vi "PLC-Connection Status.vi"(8 "error in (no error)":errorcluster, 9 "Remarks":string, 10 "Status":bool, 11 "Controller in":refnum<class "Controller.lvclass">) -> (0 "error out":errorcluster, 3 "Controller out":refnum<class "Controller.lvclass">)   [LabVIEW 2021, in "Controller.lvlib" / "Controller.lvclass"]
uses:
  Controller.lvclass
  UserInterface/UserInterface Messages/PLC Status Msg/PLC Status Msg.lvclass
  UserInterface/UserInterface Messages/Log Data Msg/Log Data Msg.lvclass
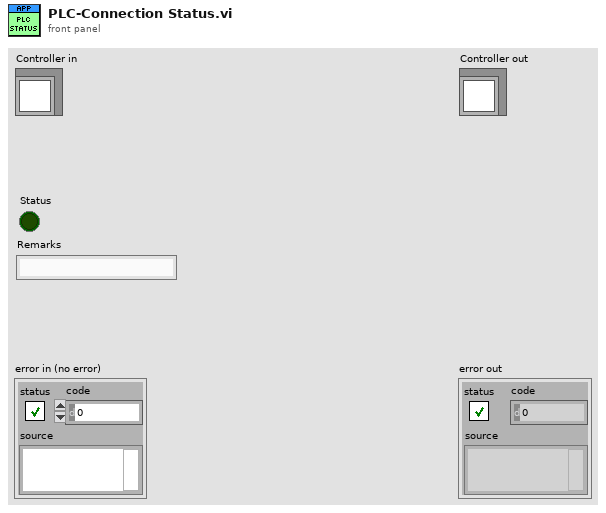
[diagram p1: front panel]
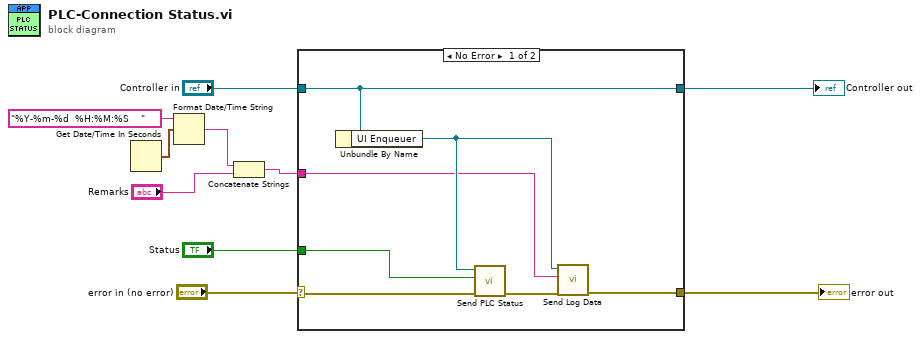
[diagram p0: block diagram]
diagram:
  n1 = Get Date/Time In Seconds() -> (seconds since 1Jan1904=w2:timestamp)
  n2 = Format Date/Time String(time format string (%c)="%Y-%m-%d  %H:%M:%S    ", seconds (now)=w2) -> (date/time string=w1:string)  [unwired: 1 in]
  n3 = Concatenate Strings(w1, "Remarks") -> (w4:string)
  n4 = case shown="No Error" "error in (no error)" {
    selector: "error in (no error)" -> [w13 w18]
    tunnel: [w17 w18] -> w10
    tunnel: "Controller in" -> [w11 w19]
    tunnel: "Status" -> [w16 _]
    tunnel: w4 -> [w12 _]
    tunnel: [w11 w19] -> w5
    frame No Error {
      n5 = Unbundle By Name(w11) -> ("UI Enqueuer"=w14:refnum<class "Message Enqueuer.lvclass">)
      n6 = call "Send PLC Status.vi"("error in (no error)"=w13, "PLC Status"=w16, "Message Enqueuer"=w14) -> ("error out"=w15:errorcluster)  [unwired: 7 in, 1 out]
      n7 = call "Send Log Data.vi"("error in (no error)"=w15, "Message"=w12, "Message Enqueuer"=w14) -> ("error out"=w17:errorcluster)  [unwired: 7 in, 1 out]
    }
    frame Error {
    }
  }
  "error out" <- w10
  "Controller out" <- w5
